vi "Write ExplicitFieldOrder.vi"(8 "error in (no error)":errorcluster, 10 "ExplicitFieldOrder":string[](array[string]), 11 "TypeMap in":refnum<class "TypeMap.lvclass">) -> (0 "error out":errorcluster, 3 "TypeMap out":refnum<class "TypeMap.lvclass">)   [LabVIEW 2020, in "ORM.lvlib" / "TypeMap.lvclass"]
uses:
  TypeMap.lvclass
  TypeMap.lvclass/TypeMap.ctl
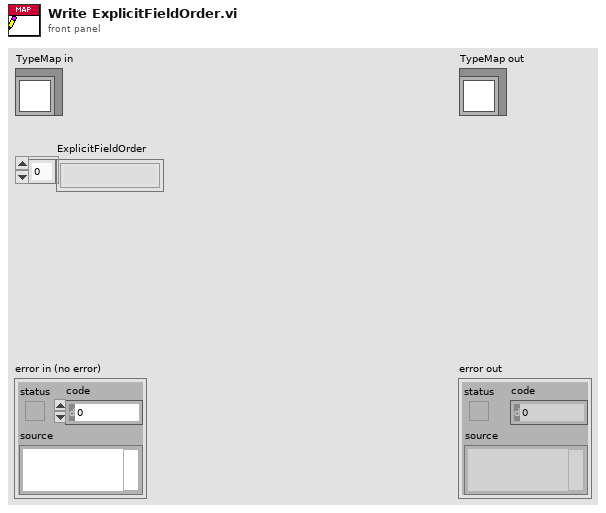
[diagram p1: front panel]
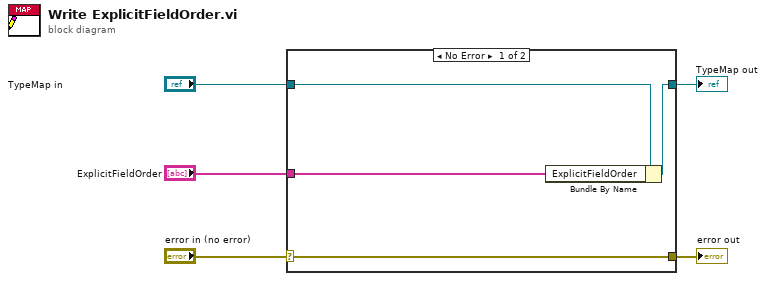
[diagram p0: block diagram]
diagram:
  n1 = case shown="No Error" "error in (no error)" {
    selector: "error in (no error)" -> [w9 w10]
    tunnel: [w9 w10] -> w4
    tunnel: [w7 w11] -> w2
    tunnel: "TypeMap in" -> [w8 w11]
    tunnel: "ExplicitFieldOrder" -> [w6 _]
    frame No Error {
      n2 = Bundle By Name(cluster=w8, "ExplicitFieldOrder"=w6) -> (w7:refnum<class "TypeMap.lvclass">)
    }
    frame Error {
    }
  }
  "error out" <- w4
  "TypeMap out" <- w2
